vi "rsp_Connection Lost.vi"(8 "error in":errorcluster, 9 "Data in":T1, 11 "DS TCP Read in":refnum<class "DS TCP Read.lvclass">) -> (0 "error out":errorcluster, 3 "dup DS TCP Read out":refnum<class "DS TCP Read.lvclass">)   [LabVIEW 2017, in "DS TCP Server.lvlib" / "DS TCP Read.lvclass"]
doc: "This VI sends a <b>Public API Response</b> message to a registered MHL case of the Caller of the Worker that owns this VI.\n---"
uses:
  DS TCP Read.lvclass
  C:/Program Files (x86)/National Instruments/LabVIEW 2017/vi.lib/addons/_Workers/Library/Classes/Worker/Worker.lvclass
  rsp_Connection Lost.ctl
  <vilib>/addons/_Workers/Library/Classes/Message Queue/Message Queue.lvclass
  DS TCP Read.lvclass/DS TCP Read.ctl
  <vilib>/addons/_Workers/Library/Classes/Worker/Worker.lvclass/Worker.ctl
  <vilib>/addons/_Workers/Library/Classes/Message/Priority.ctl
  <vilib>/Utility/error.llb/Error Cluster From Error Code.vi
  <vilib>/addons/_Workers/Library/Classes/Message/Enqueue Message to Queue.vi
  <vilib>/ErrorRing/Error Ring.xnode
  <vilib>/addons/_Workers/Library/Classes/Message/Message.lvclass
  <vilib>/addons/_Workers/Library/Classes/Worker/Worker.lvclass
  C:/Program Files (x86)/National Instruments/LabVIEW 2017/vi.lib/addons/_Workers/Library/Classes/Workers Object/Workers Object.lvclass
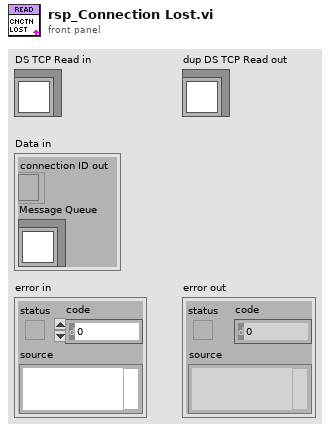
[diagram p1: front panel]
types:
  T1 = typedef "DS TCP Server.lvlib/DS TCP Read.lvclass/rsp_Connection Lost.ctl" = cluster{"connection ID out":refnum<k5>, "Message Queue":refnum<class "Message Queue.lvclass">}
  T2 = typedef "Workers.lvlib/Case Label.ctl" = string
  T3 = typedef "Workers.lvlib/Message.lvclass/Priority.ctl" = enum16{"Low", "Normal", "High"}
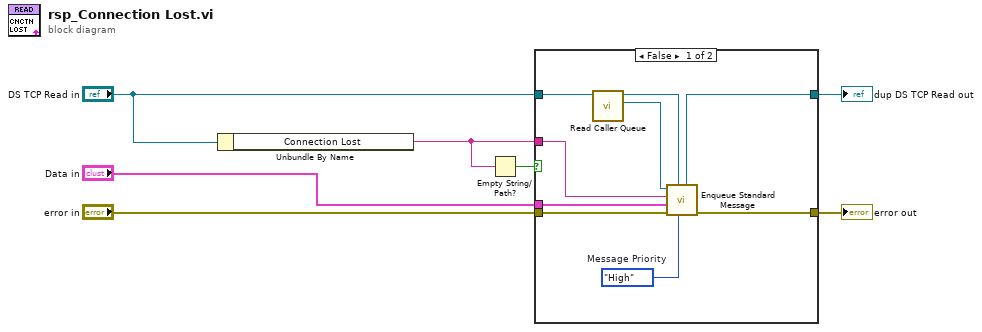
[diagram p0: block diagram]
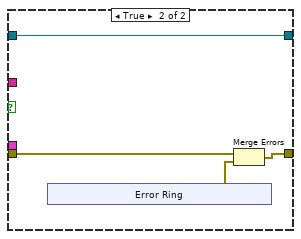
[diagram p2: hidden frame]
diagram:
  n1 = Unbundle By Name("DS TCP Read in") -> ("Connection Lost"=w2:T2)
  n2 = Empty String/Path?(string/path=w2) -> (empty?=w3:bool)
  n3 = case shown="False" w3 {
    tunnel: "error in" -> [w10 w17]
    tunnel: [w16 w18] -> w6
    tunnel: "Data in" -> [w14 _]
    tunnel: [w13 w20] -> w4
    tunnel: "DS TCP Read in" -> [w11 w20]
    tunnel: w2 -> [w12 _]
    frame False {
      w15 = Priority."High"  # Message Priority
      n4 = call <vilib>:"Read Caller Queue.vi"("Worker_"=w11) -> ("Message Queue out"=w8:refnum<class "Message Queue.lvclass">, "dup Worker_out"=w9:refnum<class "DS TCP Read.lvclass">)  [unwired: 9 in]
      n5 = call-poly <vilib>:"Enqueue Standard Message.vi"("Priority (Normal)"=w15, "Worker"=w9, "error in"=w10, "Data"=w14, "Case Label"=w12, "Message Queue"=w8) -> ("error out"=w16:errorcluster, "dup Worker out"=w13:refnum<class "DS TCP Read.lvclass">)  [unwired: 3 in, 1 out]
    }
    frame True {
      n6 = xnode "Error Ring"() -> ("error out"=w19:errorcluster)
      n7 = Merge Errors(w17, w19) -> (w18:errorcluster)
    }
  }
  "error out" <- w6
  "dup DS TCP Read out" <- w4
